vi "SSL Tester.vi"() -> ()   [LabVIEW 2015, in "AWS_IoT.lvlib"]
uses:
  AWS_IoT.lvlib
  Controls/SSL_Connection.ctl
  Controls/SSL_login.ctl
  Controls/certs.ctl
panel:
  in  "certs":T1={"client cert file"=path "", "CA file"=path "", "client key file"=path ""}
  out "timeout?":bool
  out "data out 2":u8[](array[numeric]) format="%x"
  in  "login":T2={"server IP"="", "server port"=0, "local port (0 = auto)"=0, "timeout ms (1000)"=1000}
  out "error out":errorcluster
  out "data out":u8[](array[numeric]) format="%x"
  in  "SSL_Connection":T3
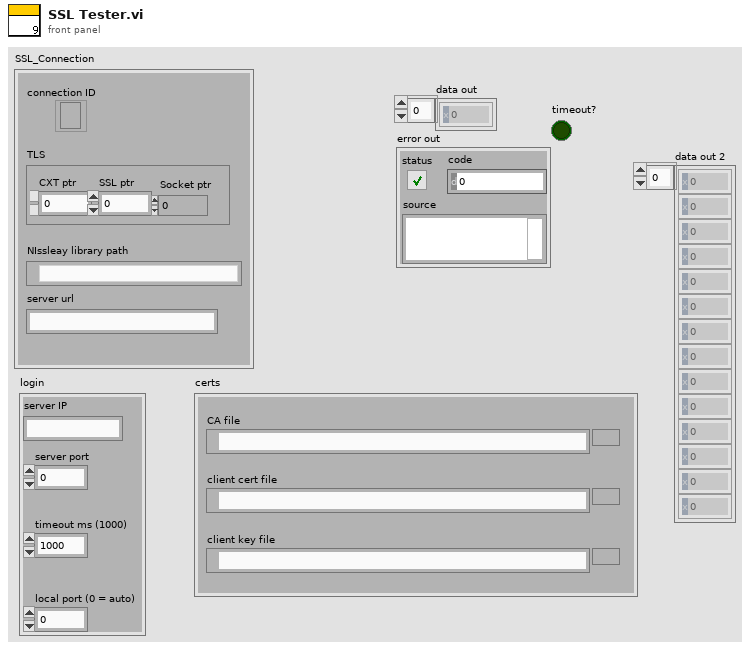
[diagram p1: front panel]
types:
  T1 = typedef "AWS_IoT.lvlib/certs.ctl" = cluster{"client cert file":path, "CA file":path, "client key file":path}
  T2 = typedef "AWS_IoT.lvlib/SSL_login.ctl" = cluster{"server IP":string, "server port":u16, "local port (0 = auto)":u16, "timeout ms (1000)":i32}
  T3 = typedef "AWS_IoT.lvlib/SSL_Connection.ctl" = cluster{"connection ID":refnum<k5>, "TLS":cluster{"CXT ptr":i32, "SSL ptr":i32, "Socket ptr":i32}, "NIssleay library path":path, "server url":string}
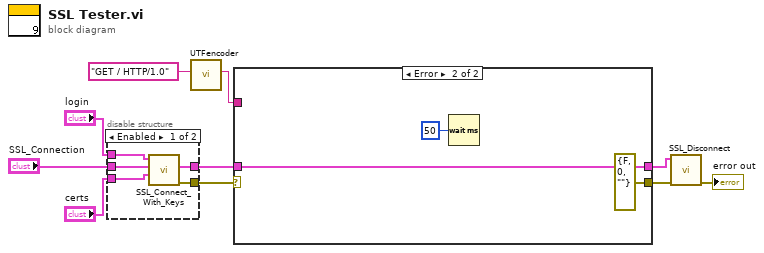
[diagram p0: block diagram]
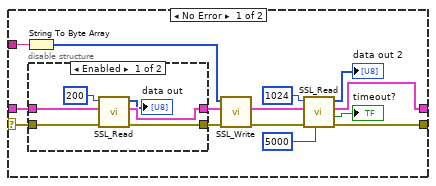
[diagram p2: hidden frame]
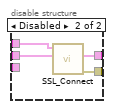
[diagram p4: hidden frame]
diagram:
  n1 = disable-structure shown="Enabled" {
    disable-tunnel: [w15 w17] -> w10
    disable-tunnel: [w14 w16] -> w1
    disable-tunnel: "SSL_Connection" -> [w13 w18]
    disable-tunnel: "login" -> [w12 w19]
    disable-tunnel: "certs" -> [w11 _]
    frame Enabled {
      n2 = call "SSL_Connect_With_Keys.vi"("cert path"=w11, "SSL_Connection"=w13, "login"=w12) -> ("error out"=w14:errorcluster, "SSL_Connection"=w15:T3)  [unwired: 7 in]
    }
    frame Disabled {
      n3 = call "SSL_Connect.vi"("SSL_Connection"=w18, "login"=w19) -> ("error out"=w16:errorcluster, "SSL_Connection"=w17:T3)  [unwired: 8 in]
    }
  }
  n4 = call "UTFencoder.vi"("LabVIEW string"="GET / HTTP/1.0") -> ("UTF-8 string"=w3:string)  [unwired: 10 in]
  n5 = case shown="Error" w1 {
    selector: w1 -> [w20 _]
    tunnel: w10 -> [w33 w44]
    tunnel: [w27 errorcluster {"status"=FALSE, "code"=0, "source"=""} ("error out")] -> w6
    tunnel: [w26 w44] -> w5
    tunnel: w3 -> [w21 _]
    frame No Error {
      n6 = String To Byte Array(string=w21) -> (unsigned byte array=w30:u8[])
      n7 = disable-structure shown="Enabled" {
        disable-tunnel: w33 -> [w39 w41]
        disable-tunnel: w20 -> [w37 w40]
        disable-tunnel: [w36 w40] -> w32
        disable-tunnel: [w35 w41] -> w31
        frame Enabled {
          n8 = call "SSL_Read.vi"("error in (no error)"=w37, "SSL_Connection"=w39, "bytes to read"=200) -> ("error out"=w36:errorcluster, "SSL_Connection 2"=w35:T3, "data out"=→"data out":u8[])  [unwired: 5 in, 1 out]
        }
        frame Disabled {
        }
      }
      n9 = call "SSL_Write.vi"("error in (no error)"=w32, "SSL_Connection"=w31, "data in"=w30) -> ("error out"=w28:errorcluster, "SSL_Connection"=w29:T3)  [unwired: 7 in]
      n10 = call "SSL_Read.vi"("timeout ms (5000)"=5000, "error in (no error)"=w28, "SSL_Connection"=w29, "bytes to read"=1024) -> ("error out"=w27:errorcluster, "timeout?"=→"timeout?":bool, "SSL_Connection 2"=w26:T3, "data out"=→"data out 2":u8[])  [unwired: 4 in]
    }
    frame Error {
      n11 = Wait (ms)(milliseconds to wait=u32 50) -> ()  [unwired: 1 out]
    }
  }
  n12 = call "SSL_Disconnect.vi"("error in (no error)"=w6, "SSL_Connection"=w5) -> ("error out"=→"error out":errorcluster)  [unwired: 9 in]
